vi "main.vi"() -> ()   [LabVIEW 2023]
uses:
  <vilib>/Utility/file.llb/Read Delimited Spreadsheet (string).vi
  Global 1.vi
panel:
  in  "stop":bool
  in  "Client_btn":bool caption="Operator_btn"
  in  "Service_btn":bool caption="Operator_btn"
  in  "Operator_btn":bool
  # "Log into the system as:"
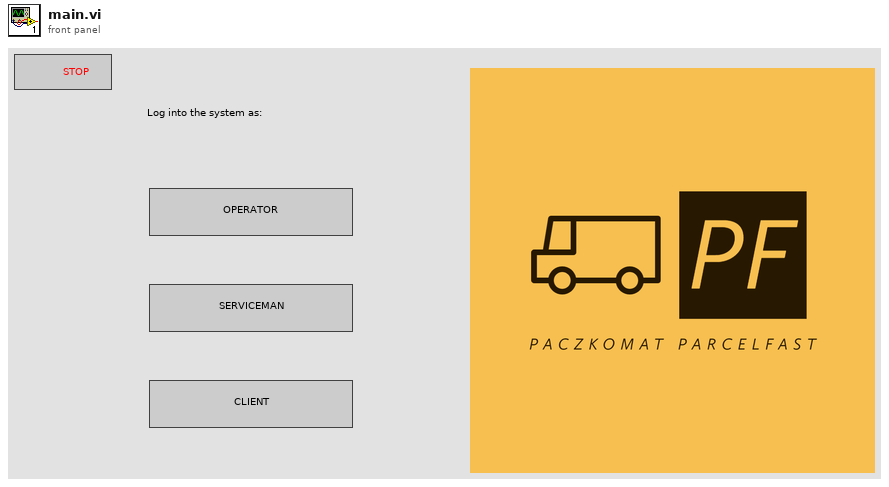
[diagram p1: front panel]
types:
  T1 = cluster{"operator":bool, "serviceman":bool, "user":bool}
  T2 = enum32{"Bad", "Idle", "Run top level", "Running"}
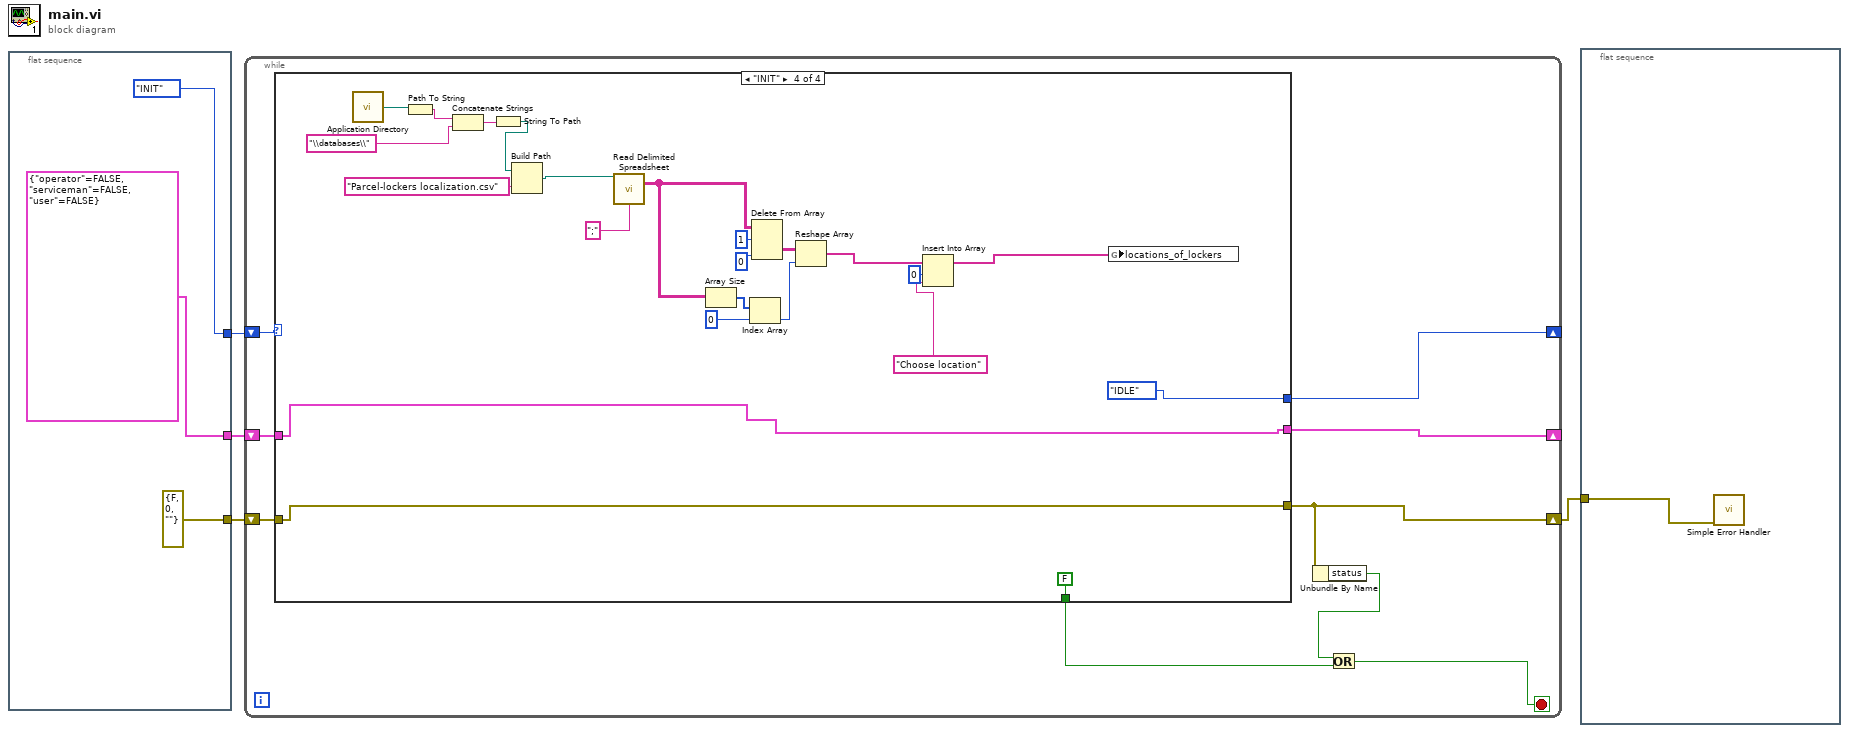
[diagram p0: block diagram]
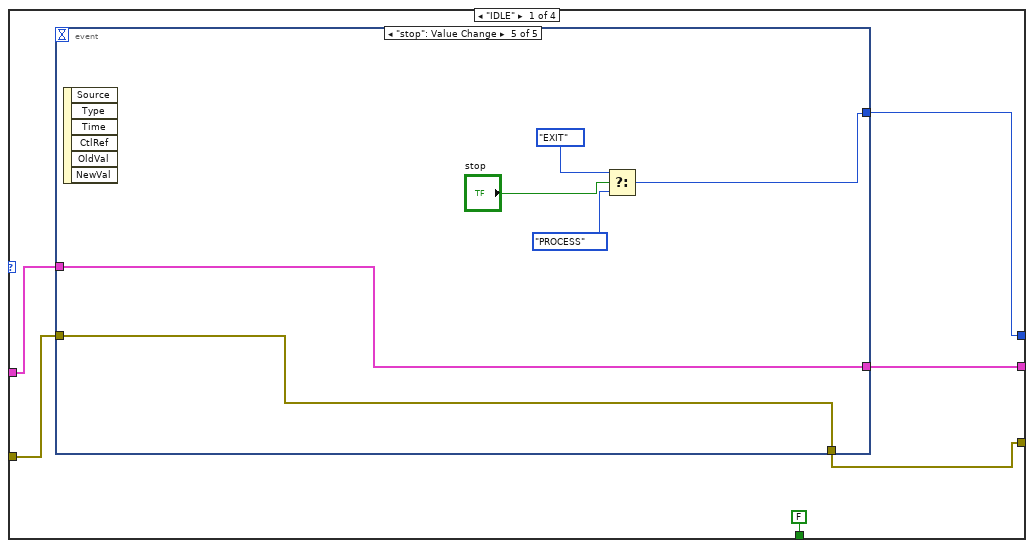
[diagram p2: hidden frame]
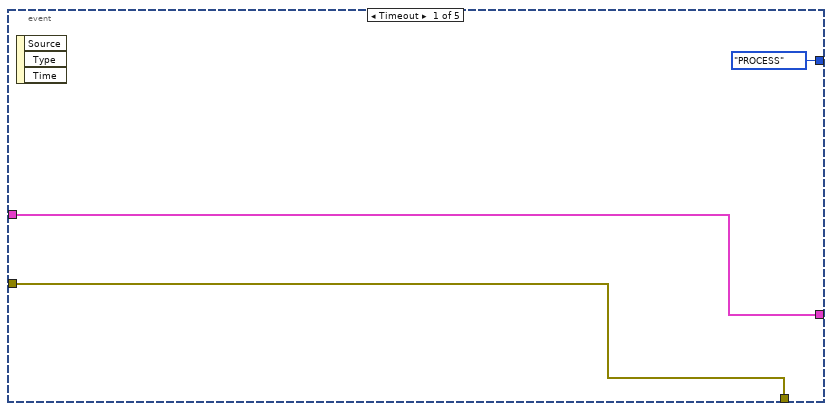
[diagram p3: hidden frame]
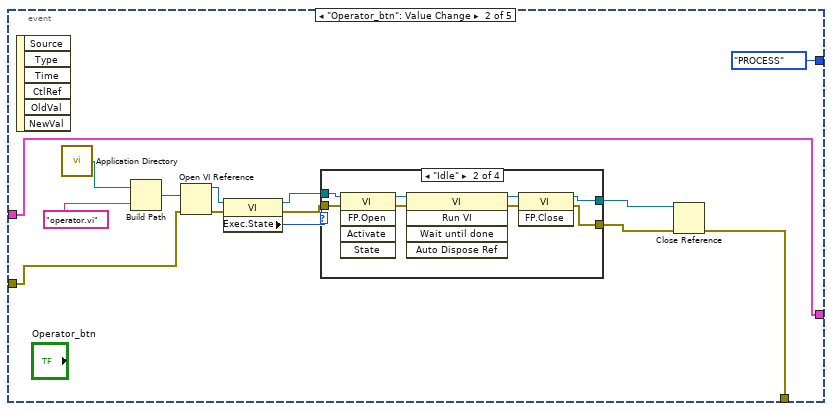
[diagram p4: hidden frame]
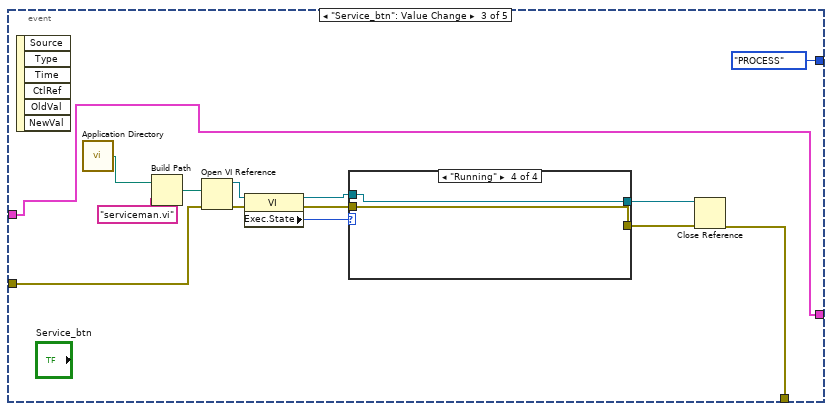
[diagram p8: hidden frame]
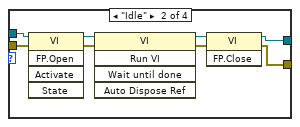
[diagram p10: hidden frame]
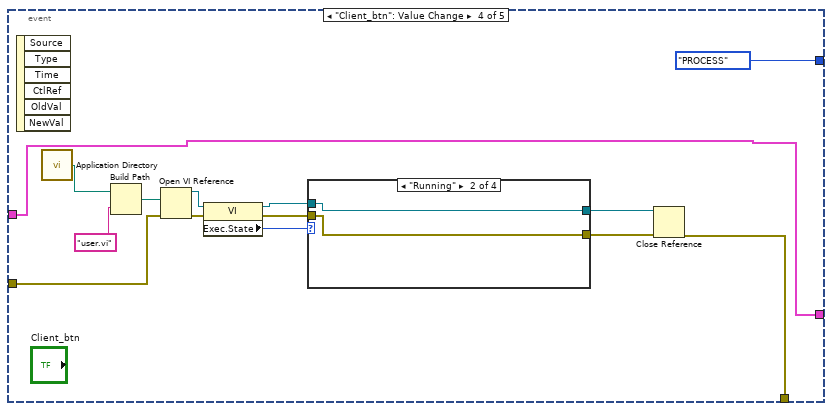
[diagram p12: hidden frame]
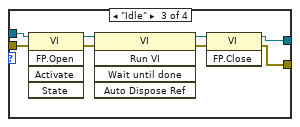
[diagram p14: hidden frame]
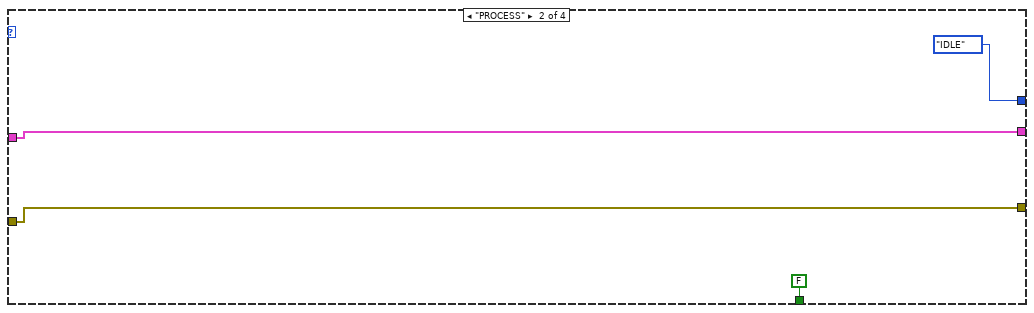
[diagram p16: hidden frame]
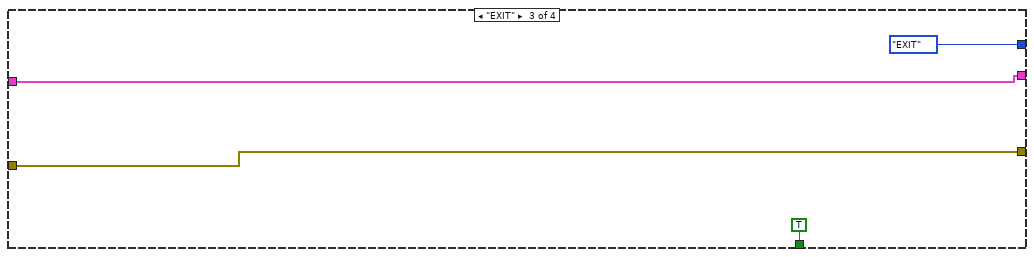
[diagram p17: hidden frame]
diagram:
  n1 = flat-sequence {
    tunnel: [enum16{"INIT", "IDLE", "PROCESS", "EXIT"}."INIT"] -> w4
    tunnel: [errorcluster {"status"=FALSE, "code"=0, "source"=""} ("error constant")] -> w2
    tunnel: [T1 {"operator"=FALSE, "serviceman"=FALSE, "user"=FALSE}] -> w1
    frame #0 {
    }
  }
  n2 = while {
    shift-right: [w16] -> _
    shift-left: w4 -> [w8]
    shift-right: [w13] -> w3
    shift-left: w2 -> [w15]
    shift-right: [w10] -> _
    shift-left: w1 -> [w9]
    stop <- w11 stop-if-true
    n3 = case shown="\"INIT\"" w8 {
      tunnel: [FALSE ("stop") FALSE ("stop") TRUE ("stop") FALSE ("stop")] -> w14
      tunnel: w9 -> [w20 w119 w120 w143]
      tunnel: [w17 enum16{"INIT", "IDLE", "PROCESS", "EXIT"}."IDLE" ("f") enum16{"INIT", "IDLE", "PROCESS", "EXIT"}."EXIT" enum16{"INIT", "IDLE", "PROCESS", "EXIT"}."IDLE"] -> w16
      tunnel: [w18 w117 w121 w144] -> w13
      tunnel: w15 -> [w19 w117 w121 w144]
      tunnel: [w21 w119 w120 w143] -> w10
      frame "IDLE" {
        n4 = event shown="[4] \"stop\": Value Change" {
          selector: _ -> [_ _ _ _ _]
          dyn-events: _ -> [_ _ _ _ _]
          timeout: _ -> [_ _ _ _ _]
          tunnel: [w25 w33 w55 w84 w115] -> w21
          tunnel: w20 -> [w25 w33 w55 w84 w115]
          tunnel: w19 -> [w24 w32 w57 w83 w114]
          tunnel: [w24 w34 w56 w85 w114] -> w18
          tunnel: [enum16{"INIT", "IDLE", "PROCESS", "EXIT"}."PROCESS" ("f") enum16{"INIT", "IDLE", "PROCESS", "EXIT"}."PROCESS" ("f") enum16{"INIT", "IDLE", "PROCESS", "EXIT"}."PROCESS" ("f") enum16{"INIT", "IDLE", "PROCESS", "EXIT"}."PROCESS" w110] -> w17
          event Timeout {
            n5 = event-data() -> ()  [unwired: 1 in, 3 out]
          }
          event "Operator_btn": Value Change {
            n6 = event-data() -> ()  [unwired: 1 in, 6 out]
            n7 = call <vilib>:"Application Directory.vi"() -> ("Application Directory"=w39:path)
            n8 = Build Path(base path=w39, name or relative path="operator.vi") -> (appended path=w37:path)
            n9 = Open VI Reference(vi path=w37, error in (no error)=w32) -> (vi reference=w36:refnum<vi>, error out=w35:errorcluster)  [unwired: 4 in]
            n10 = property class="VI"(reference=w36, error in=w35) -> (reference out=w30:refnum<vi>, error out=w29:errorcluster, "Exec.State"=w28:T2)
            n11 = case shown="\"Idle\"" w28 {
              tunnel: w30 -> [w41 w49 w51 w53]
              tunnel: w29 -> [w40 w48 w50 w52]
              tunnel: [w41 w43 w51 w53] -> w27
              tunnel: [w40 w42 w50 w52] -> w26
              frame "Bad", Default {
              }
              frame "Idle" {
                n12 = invoke class="VI" method="FP.Open"(reference=w49, error in=w48) -> (reference out=w47:refnum<vi>, error out=w46:errorcluster)  [unwired: 3 in, 3 out]
                n13 = invoke class="VI" method="Run VI"(reference=w47, error in=w46) -> (reference out=w45:refnum<vi>, error out=w44:errorcluster)  [unwired: 3 in, 3 out]
                n14 = invoke class="VI" method="FP.Close"(reference=w45, error in=w44) -> (reference out=w43:refnum<vi>, error out=w42:errorcluster)  [unwired: 1 in, 1 out]
              }
              frame "Run top level" {
              }
              frame "Running" {
              }
            }
            n15 = Close Reference(reference=w27, error in (no error)=w26) -> (error out=w34:errorcluster)
          }
          event "Service_btn": Value Change {
            n16 = event-data() -> ()  [unwired: 1 in, 6 out]
            n17 = call <vilib>:"Application Directory.vi"() -> ("Application Directory"=w67:path)
            n18 = Build Path(base path=w67, name or relative path="serviceman.vi") -> (appended path=w66:path)
            n19 = Open VI Reference(vi path=w66, error in (no error)=w57) -> (vi reference=w65:refnum<vi>, error out=w64:errorcluster)  [unwired: 4 in]
            n20 = property class="VI"(reference=w65, error in=w64) -> (reference out=w62:refnum<vi>, error out=w61:errorcluster, "Exec.State"=w63:T2)
            n21 = case shown="\"Running\"" w63 {
              tunnel: w62 -> [w69 w77 w79 w81]
              tunnel: w61 -> [w68 w76 w78 w80]
              tunnel: [w69 w71 w79 w81] -> w60
              tunnel: [w68 w70 w78 w80] -> w59
              frame "Bad", Default {
              }
              frame "Idle" {
                n22 = invoke class="VI" method="FP.Open"(reference=w77, error in=w76) -> (reference out=w75:refnum<vi>, error out=w74:errorcluster)  [unwired: 3 in, 3 out]
                n23 = invoke class="VI" method="Run VI"(reference=w75, error in=w74) -> (reference out=w73:refnum<vi>, error out=w72:errorcluster)  [unwired: 3 in, 3 out]
                n24 = invoke class="VI" method="FP.Close"(reference=w73, error in=w72) -> (reference out=w71:refnum<vi>, error out=w70:errorcluster)  [unwired: 1 in, 1 out]
              }
              frame "Run top level" {
              }
              frame "Running" {
              }
            }
            n25 = Close Reference(reference=w60, error in (no error)=w59) -> (error out=w56:errorcluster)
          }
          event "Client_btn": Value Change {
            n26 = event-data() -> ()  [unwired: 1 in, 6 out]
            n27 = call <vilib>:"Application Directory.vi"() -> ("Application Directory"=w95:path)
            n28 = Build Path(base path=w95, name or relative path="user.vi") -> (appended path=w94:path)
            n29 = Open VI Reference(vi path=w94, error in (no error)=w83) -> (vi reference=w93:refnum<vi>, error out=w92:errorcluster)  [unwired: 4 in]
            n30 = property class="VI"(reference=w93, error in=w92) -> (reference out=w90:refnum<vi>, error out=w89:errorcluster, "Exec.State"=w91:T2)
            n31 = case shown="\"Running\"" w91 {
              tunnel: w90 -> [w97 w99 w107 w109]
              tunnel: w89 -> [w96 w98 w106 w108]
              tunnel: [w97 w99 w101 w109] -> w88
              tunnel: [w96 w98 w100 w108] -> w87
              frame "Bad", Default {
              }
              frame "Running" {
              }
              frame "Idle" {
                n32 = invoke class="VI" method="FP.Open"(reference=w107, error in=w106) -> (reference out=w105:refnum<vi>, error out=w104:errorcluster)  [unwired: 3 in, 3 out]
                n33 = invoke class="VI" method="Run VI"(reference=w105, error in=w104) -> (reference out=w103:refnum<vi>, error out=w102:errorcluster)  [unwired: 3 in, 3 out]
                n34 = invoke class="VI" method="FP.Close"(reference=w103, error in=w102) -> (reference out=w101:refnum<vi>, error out=w100:errorcluster)  [unwired: 1 in, 1 out]
              }
              frame "Run top level" {
              }
            }
            n35 = Close Reference(reference=w88, error in (no error)=w87) -> (error out=w85:errorcluster)
          }
          event "stop": Value Change {
            n36 = event-data() -> ()  [unwired: 1 in, 6 out]
            n37 = Select(t=enum16{"INIT", "IDLE", "PROCESS", "EXIT"}."EXIT", s="stop", f=enum16{"INIT", "IDLE", "PROCESS", "EXIT"}."PROCESS") -> (s? t:f=w110:enum16{"INIT", "IDLE", "PROCESS", "EXIT"})
          }
        }
      }
      frame "PROCESS" {
      }
      frame "EXIT" {
      }
      frame "INIT" {
        n38 = call <vilib>:"Application Directory.vi"() -> ("Application Directory"=w141:path)
        n39 = Path To String(path=w141) -> (string=w140:string)
        n40 = Concatenate Strings(w140, "\\databases\\") -> (w138:string)
        n41 = String To Path(string=w138) -> (path=w137:path)
        n42 = Build Path(base path=w137, name or relative path="Parcel-lockers localization.csv") -> (appended path=w135:path)
        n43 = call-poly <vilib>:"Read Delimited Spreadsheet.vi"("file path (dialog if empty)"=w135, "delimiter (\\t)"=";" ("delimiter (\\t)")) -> ("all rows"=w131:string[][])  [unwired: 8 in, 5 out]
        n44 = Array Size(array=w131) -> (size(s)=w130:i32[])
        n45 = Index Array "Index Array"(array=w130, index=0) -> (element=w128:i32)
        n46 = Delete From Array(array=w131, length=1, index (col)=0 ("disabled index (col)")) -> (deleted portion=w132:string[][])  [unwired: 1 in, 1 out]
        n47 = Reshape Array(w132, w128) -> (w127:string[])
        n48 = Insert Into Array "Insert Into Array"(array=w127, index=0, new element="Choose location" ("new element/subarray")) -> (w124:string[])
        n49 = global write "Global 1.vi" "locations_of_lockers"(w124) -> ()
      }
    }
    n50 = Unbundle By Name(w13) -> ("status"=w12:bool)
    n51 = Or(x=w12, y=w14) -> (x .or. y?=w11:bool)
  }
  n52 = flat-sequence {
    tunnel: w3 -> [w147]
    frame #0 {
      n53 = call <vilib>:"Simple Error Handler.vi"("error in (no error)"=w147) -> ()  [unwired: 4 in, 5 out]
    }
  }
